vi "testCheckQueueFull.vi"(8 "error in (no error)":errorcluster) -> (0 "error out":errorcluster)   [LabVIEW 2018]
doc: "Test the checkQueueFull.vi."
uses:
  src/TcpServer/TcpServer.lvclass
  src/TcpServerTel/typedef/enqueueOptionsTypeDef.ctl
  src/TcpServerTel/typedef/queueOptionsTypeDef.ctl
  src/TcpServer/TcpServer.lvclass/TcpServer.ctl
  src/TcpServerTel/typedef/telTypeDef.ctl
  src/TcpServerBase/TcpServerBase.lvclass/TcpServerBase.ctl
  src/TcpServerTel/TcpServerTel.lvclass
  home/pcortes/github/ts_labview_tcp_json/src/TcpServerBase/TcpServerBase.lvclass
  <vilib>/addons/_JKI Toolkits/Caraya/classes/Assert/Assert False.vi
  <vilib>/addons/_JKI Toolkits/Caraya/classes/Assert/Assert True.vi
  <vilib>/addons/_JKI Toolkits/Caraya/classes/Test/Test.lvclass
  <vilib>/addons/_JKI Toolkits/Caraya/classes/Assert/Assert.lvclass
  src/TcpServerBase/TcpServerBase.lvclass
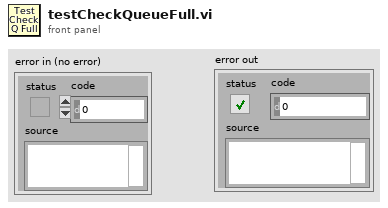
[diagram p1: front panel]
types:
  T1 = typedef "TcpServerTel.lvclass/enqueueOptionsTypeDef.ctl" = enum16{"lossy enqueue", "normal enqueue"}
  T2 = typedef "TcpServerTel.lvclass/queueOptionsTypeDef.ctl" = cluster{"EnqueueOptions":T1, "Timeout (ms)":i32}
  T3 = cluster{"cmdServerPort":u16, "telServerPort":u16, "serverTimeout (ms)":i32, "serverBytesToRead":i32, "telQueueServerMaxSize":i32, "EnqueueOptions":T1, "telQueueServerTimeout":i32, "tcpClientQueueMaxSize":i32}
  T4 = typedef "TcpServerTel.lvclass/telTypeDef.ctl" = cluster{"name":string, "telDetails":string}
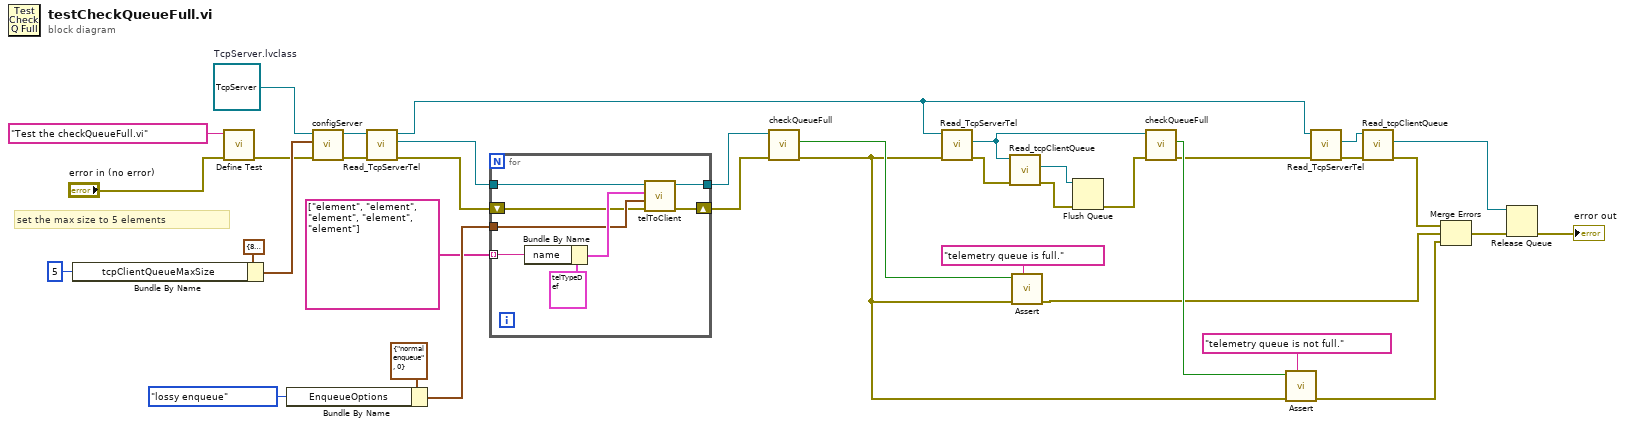
[diagram p0: block diagram]
diagram:
  w25 = refnum<class "TcpServer.lvclass"> refnum  # TcpServer.lvclass
  # "set the max size to 5 elements"
  n1 = Bundle By Name(cluster=T3 {"cmdServerPort"=8888, "telServerPort"=8888, "serverTimeout (ms)"=100, "serverBytesToRead"=32768, "telQueueServerMaxSize"=1000, "EnqueueOptions"=enum."lossy enqueue", "telQueueServerTimeout"=50, "tcpClientQueueMaxSize"=100} ("ServerConfiguration"), "tcpClientQueueMaxSize"=5 ("telQueueServerMaxSize")) -> (w24:T3)
  n2 = call <vilib>:"Define Test.vi"("error in (no error)"="error in (no error)", "Label (VI Title)"="Test the checkQueueFull.vi") -> ("error out"=w23:errorcluster)  [unwired: 9 in]
  n3 = Bundle By Name(cluster=T2 {"EnqueueOptions"=enum."normal enqueue", "Timeout (ms)"=0} ("queueOptions"), "EnqueueOptions"=enqueueOptionsTypeDef."lossy enqueue") -> (w16:T2)
  n4 = call "configServer.vi"("error in (no error)"=w23, "ServerConfiguration"=w24, "tcpServer in"=w25) -> ("error out"=w21:errorcluster, "tcpServer out"=w22:refnum<class "TcpServer.lvclass">)  [unwired: 7 in]
  n5 = call "Read_TcpServerTel.vi"("error in (no error)"=w21, "TcpServer in"=w22) -> ("error out"=w19:errorcluster, "TcpServerTel.lvclass"=w20:refnum<class "TcpServerTel.lvclass">, "TcpServer out"=w1:refnum<class "TcpServer.lvclass">)  [unwired: 7 in]
  n6 = for {
    tunnel: w20 -> [w45]
    tunnel: w16 -> [w41]
    shift-right: [w39] -> w15
    shift-left: w19 -> [w40]
    tunnel: string[] ["element", "element", "element", "element", "element"] -> [w43] mode=indexing
    tunnel: [w38] -> w3
    n7 = Bundle By Name(cluster=T4 {"name"="elevation", "telDetails"="\"compName\":\"MTMount\""} ("Telemetry"), "name"=w43) -> (w42:T4)
    n8 = call "telToClient.vi"("error in (no error)"=w40, "queueOptions"=w41, "Telemetry"=w42, "TcpServerTel in"=w45) -> ("error out"=w39:errorcluster, "TcpServerTel out"=w38:refnum<class "TcpServerTel.lvclass">)  [unwired: 6 in]
  }
  n9 = call "checkQueueFull.vi"("error in (no error)"=w15, "tcpServerTel in"=w3) -> ("error out"=w9:errorcluster, "isTcpClientQueueFull"=w32:bool)  [unwired: 7 in, 1 out]
  n10 = call "Read_TcpServerTel.vi"("error in (no error)"=w9, "TcpServer in"=w1) -> ("error out"=w14:errorcluster, "TcpServerTel.lvclass"=w2:refnum<class "TcpServerTel.lvclass">)  [unwired: 7 in, 1 out]
  n11 = call "Read_tcpClientQueue.vi"("error in (no error)"=w14, "TcpServerBase in"=w2) -> ("error out"=w12:errorcluster, "tcpClientQueue"=w13:refnum<queue>)  [unwired: 7 in, 1 out]
  n12 = call-poly <vilib>:"Assert.vi"("Label"="telemetry queue is full.", "error in (no error)"=w9, "True?"=w32) -> ("error out"=w6:errorcluster)  [unwired: 8 in]
  n13 = Flush Queue(queue=w13, error in (no error)=w12) -> (error out=w11:errorcluster)  [unwired: 2 out]
  n14 = call "checkQueueFull.vi"("error in (no error)"=w11, "tcpServerTel in"=w2) -> ("error out"=w7:errorcluster, "isTcpClientQueueFull"=w8:bool)  [unwired: 7 in, 1 out]
  n15 = call-poly <vilib>:"Assert.vi"("Label"="telemetry queue is not full.", "error in (no error)"=w9, "False?"=w8) -> ("error out"=w5:errorcluster)  [unwired: 8 in]
  n16 = call "Read_TcpServerTel.vi"("error in (no error)"=w7, "TcpServer in"=w1) -> ("error out"=w31:errorcluster, "TcpServerTel.lvclass"=w30:refnum<class "TcpServerTel.lvclass">)  [unwired: 7 in, 1 out]
  n17 = call "Read_tcpClientQueue.vi"("error in (no error)"=w31, "TcpServerBase in"=w30) -> ("error out"=w28:errorcluster, "tcpClientQueue"=w29:refnum<queue>)  [unwired: 7 in, 1 out]
  n18 = Merge Errors(w28, w6, w5) -> (w33:errorcluster)
  n19 = Release Queue(queue=w29, error in (no error)=w33) -> (error out=→"error out":errorcluster)  [unwired: 1 in, 2 out]
